vi "Robot Main.vi"() -> ()   [LabVIEW 2015]
doc: "Robot Main serves as the primary scheduler for your command and control robotics program. It should not be necessary to modify this VI. Instead, you should add your code to the VIs called from Robot Main - Teleop, Autonomous, and SubSystems."
uses:
  <vilib>/Rock Robotics/WPI/Camera/WPI_CameraImageSize.ctl
  Robot Type Def.ctl
  <vilib>/Rock Robotics/SystemInterfaces/NetworkCommunication/NetComm_UsageReport_ResourceType.ctl
  Framework/Robot Global Data.vi
  <vilib>/Rock Robotics/Network Tables/NT Write String.vi
panel:
  out "Application:Version Number":string
  in  "Time Stamp":timestamp
  out "Robot":T1=enum."Ghost"
  in  "error in":errorcluster
  in  "Enable LED Lights":bool
  in  "Image Size":T2=enum."320x240"
  in  "Enable Vision":bool
  in  "Finish":bool
  # "Make sure to set robot type"
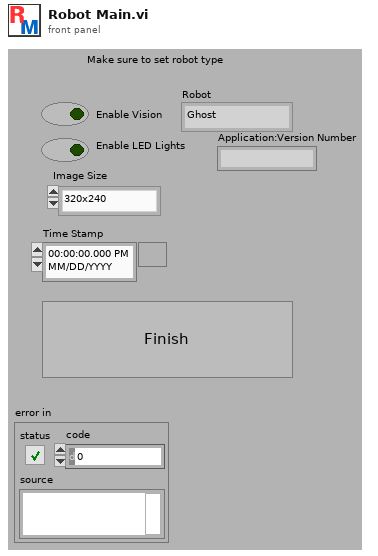
[diagram p1: front panel]
types:
  T1 = typedef "Robot Type Def.ctl" = enum32{"Disabled", "Ghost", "Casper", "Lofty", "Board", "RaceRobot"}
  T2 = typedef "WPI_CameraImageSize.ctl" = enum16{"640x480", "320x240", "160x120", "Custom"}
  T3 = typedef "NetComm_UsageReport_ResourceType.ctl" = enum8{"Controller", "Module", "Language", "CANPlugin", "Accelerometer", "ADXL345", "AnalogChannel", "AnalogTrigger", "AnalogTriggerOutput", "CANJaguar", "Compressor", "Counter", "Dashboard", "DigitalInput", "DigitalOutput", "DriverStationCIO", "DriverStationEIO", "DriverStationLCD", "Encoder", "GearTooth", "Gyro", "I2C", "Framework", "Jaguar", "Joystick", "Kinect", "KinectStick", "PIDController", "Preferences", "PWM", "Relay", "RobotDrive", "SerialPort", "Servo", "Solenoid", "SPI", "Task", "Ultrasonic", "Victor", "Button", "Command", "AxisCamera", "PCVideoServer", "SmartDashboard", "Talon", "HiTechnicColorSensor", "HiTechnicAccel", "HiTechnicCompass", "SRF08", "AnalogOutput", "Victor SP", "Talon SRX", "CAN Talon SRX", "ADXL362 Accel", "ADXRS450 Gyro", "Rev SPARK", "Mindsensors SD540", "Digital Filter"}
  T4 = typedef "WPI_DriverStationMatch Info.ctl" = cluster{"Autonomous Elapsed Seconds":dbl, "TeleOp Elapsed Seconds":dbl, "Disabled Elapsed Seconds":dbl, "Visited Autonomous":bool, "Visited TeleOp":bool, "Visited Disabled":bool, "Autonomous Settings":cluster{"Autonomous Style":enum16{"Iterative", "Independent"}, "VI Refnum":refnum<vi>}}
  T5 = typedef "WPI_DriverStationDerivedRobotMode.ctl" = enum16{"Init", "Execute", "Stop"}
  T6 = typedef "WPI_DriverStationRobotMode2.ctl" = enum16{"Autonomous Disabled", "Autonomous Enabled", "Teleop Disabled", "Teleop Enabled", "Disconnected", "Finish", "Test Disabled", "Test Enabled", "Emergency Stopped"}
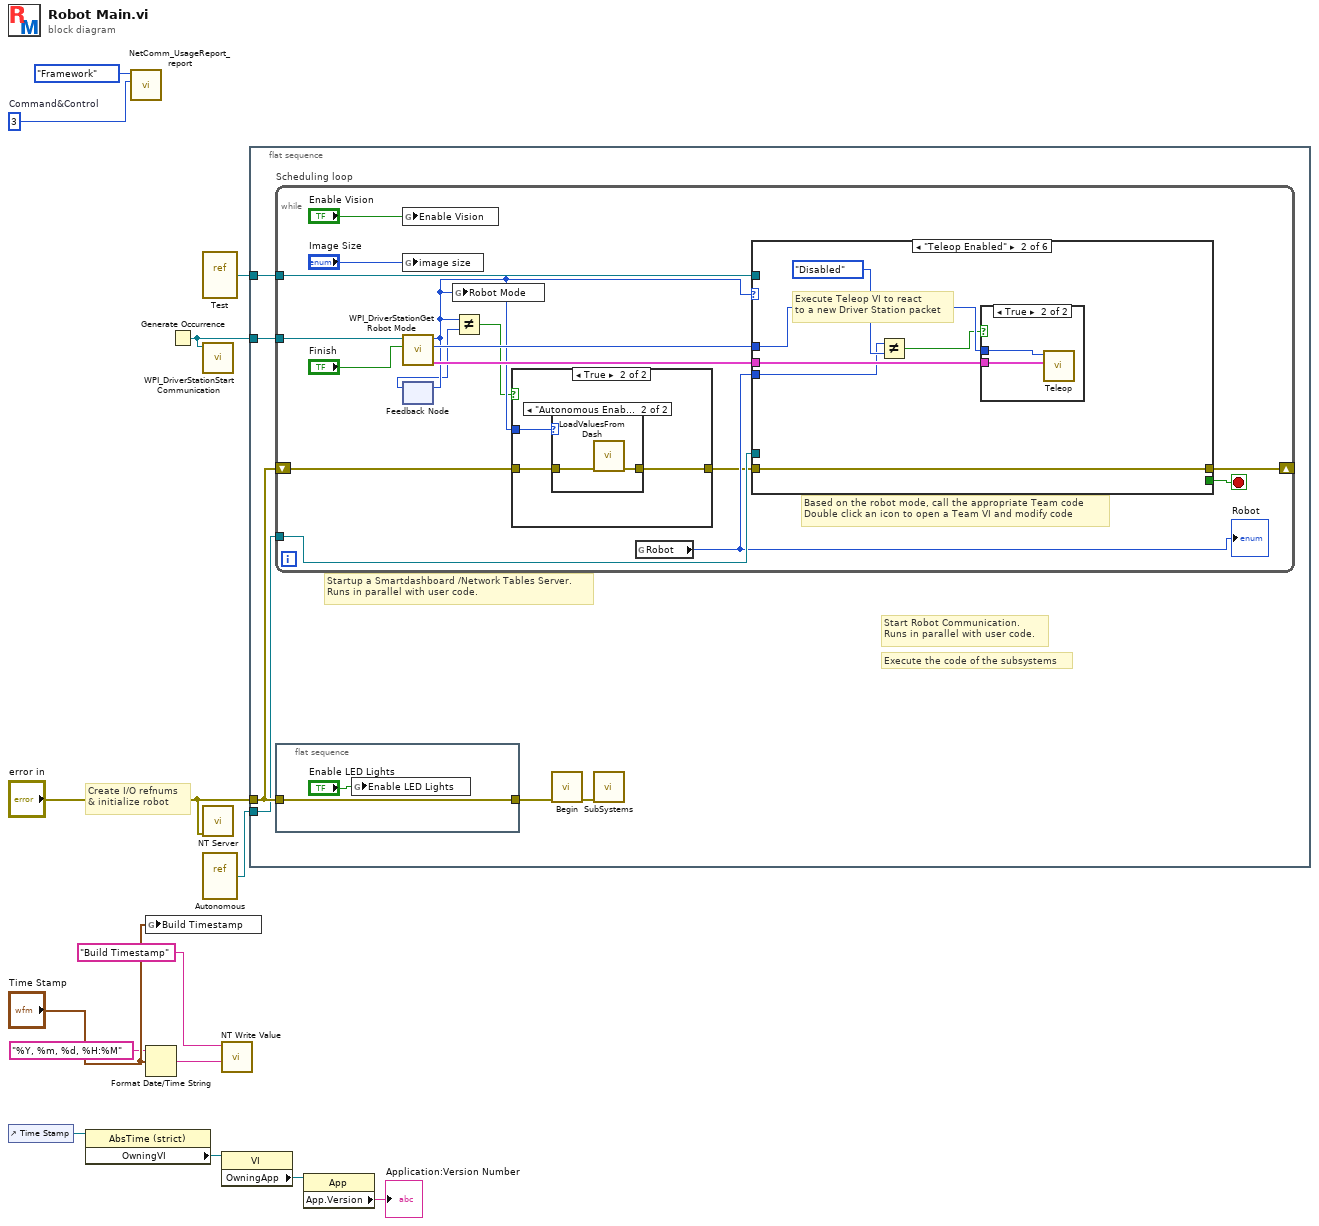
[diagram p0: block diagram]
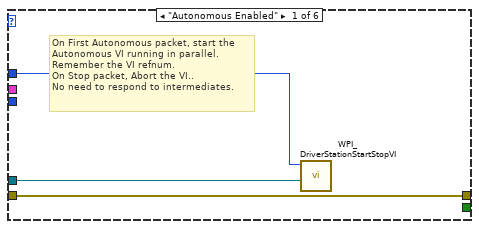
[diagram p4: hidden frame]
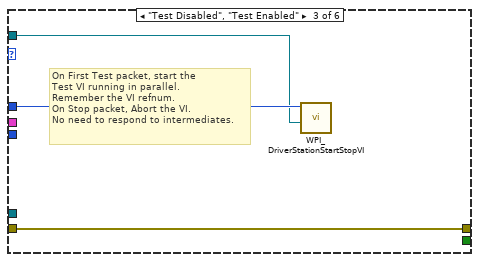
[diagram p6: hidden frame]
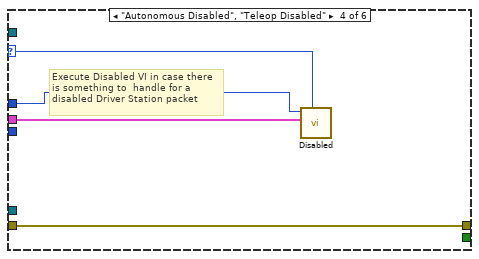
[diagram p7: hidden frame]
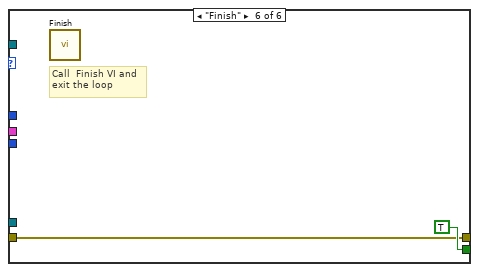
[diagram p9: hidden frame]
diagram:
  w9 = u8 3  # Command&Control
  # "Create I/O refnums\n& initialize robot"
  n1 = control-ref of="Time Stamp"() -> (w4:refnum<vi>)
  n2 = property class="AbsTime (strict)"(reference=w4) -> ("OwningVI"=w3:refnum<vi>)  [unwired: 1 in, 2 out]
  n3 = call <vilib>:"NetComm_UsageReport_report.vi"("Instance Number"=w9, "Resource Type"=NetComm_UsageReport_ResourceType."Framework") -> ()  [unwired: 10 in]
  n4 = global write "Robot Global Data.vi" "Build Timestamp"("Time Stamp") -> ()
  n5 = Format Date/Time String(time format string (%c)="%Y, %m, %d, %H:%M", seconds (now)="Time Stamp") -> (date/time string=w7:string)  [unwired: 1 in]
  n6 = Generate Occurrence() -> (w13:refnum<k4>)
  n7 = vi-ref "Test.vi"() -> (w11:refnum<vi>)
  n8 = call <vilib>:"WPI_DriverStationStart Communication.vi"("occurrence"=w13) -> ()  [unwired: 1 in, 10 out]
  n9 = call <vilib>:"NT Server.vi"("error in (no error)"="error in") -> ()  [unwired: 11 in]
  n10 = vi-ref "Autonomous.vi"() -> (w12:refnum<vi>)
  n11 = call-poly <vilib>:"NT Write Value.vi"("String"=w7, "Name"="Build Timestamp") -> ()  [unwired: 9 in, 1 out]
  n12 = property class="VI"(reference=w3) -> ("OwningApp"=w2:refnum<vi>)  [unwired: 1 in, 2 out]
  n13 = flat-sequence {
    tunnel: "error in" -> [w20]
    tunnel: w13 -> [w19]
    tunnel: w12 -> [w18]
    tunnel: w11 -> [w17]
    frame #0 {
      # "Startup a Smartdashboard /Network Tables Server.\nRuns in parallel with user code."
      # "Execute the code of the subsystems"
      # "Start Robot Communication.\nRuns in parallel with user code."
      n14 = while "Scheduling loop" {
        tunnel: w19 -> [w37]
        tunnel: w18 -> [w32]
        tunnel: w17 -> [w30]
        shift-right: [w23] -> _
        shift-left: w20 -> [w25]
        stop <- w34 stop-if-true
        # "Based on the robot mode, call the appropriate Team code\nDouble click an icon to open a Team VI and modify code"
        n15 = global write "Robot Global Data.vi" "Enable Vision"("Enable Vision") -> ()
        n16 = global write "Robot Global Data.vi" "image size"("Image Size") -> ()
        n17 = call <vilib>:"WPI_DriverStationGet Robot Mode.vi"("Finish"="Finish", "DS Occurrence"=w37) -> ("Match Info out"=w35:T4, "Call Context"=w38:T5, "Robot Mode"=w29:T6)  [unwired: 7 out]
        n18 = feedback-in #1(w29) -> ()
        n19 = feedback #1() -> (w28:T6)  [unwired: 1 in]
        n20 = global write "Robot Global Data.vi" "Robot Mode"(w29) -> ()
        n21 = Not Equal?(x=w29, y=w28) -> (x != y?=w27:bool)
        n22 = case shown="True" w27 {
          tunnel: w29 -> [_ w42]
          tunnel: w25 -> [w39 w41]
          tunnel: [w39 w40] -> w24
          frame False {
          }
          frame True {
            n23 = case shown="\"Autonomous Enabled\", \"Teleop Enabled\"" w42 {
              tunnel: w41 -> [w43 w45]
              tunnel: [w43 w44] -> w40
              frame Default {
              }
              frame "Autonomous Enabled", "Teleop Enabled" {
                n24 = call "LoadValuesFromDash.vi"("error in"=w45) -> ("error out"=w44:errorcluster)  [unwired: 10 in]
              }
            }
          }
        }
        n25 = global read "Robot Global Data.vi" "Robot"() -> (w26:T1)
        "Robot" <- w26
        n26 = case shown="\"Teleop Enabled\"" w29 {
          selector: w29 -> [_ _ _ w61 _ _]
          tunnel: w38 -> [w48 w54 w59 w63 _ _]
          tunnel: w35 -> [_ w53 _ w62 _ _]
          tunnel: [_ _ _ _ _ TRUE] -> w34
          tunnel: w32 -> [w47 _ _ _ _ _]
          tunnel: w30 -> [_ _ w58 _ _ _]
          tunnel: w26 -> [_ w50 _ _ _ _]
          tunnel: w24 -> [w46 w49 w57 w60 w64 w65]
          tunnel: [w46 w49 w57 w60 w64 w65] -> w23
          frame "Autonomous Enabled" {
            # "On First Autonomous packet, start the\nAutonomous VI running in parallel.\nRemember the VI refnum.\nOn Stop packet, Abort the VI..\nNo need to respond to intermediates."
            n27 = call <vilib>:"WPI_DriverStationStartStopVI.vi"("VI in"=w47, "Call Context"=w48) -> ()  [unwired: 10 in]
          }
          frame "Teleop Enabled" {
            # "Execute Teleop VI to react\nto a new Driver Station packet"
            n28 = Not Equal?(x=w50, y=Robot_Type_Def."Disabled" ("Robot")) -> (x != y?=w52:bool)
            n29 = case shown="True" w52 {
              tunnel: w54 -> [_ w56]
              tunnel: w53 -> [_ w55]
              frame False {
              }
              frame True {
                n30 = call "Teleop.vi"("Match Info"=w55, "Call Context"=w56) -> ()  [unwired: 1 in, 9 out]
              }
            }
          }
          frame "Test Disabled", "Test Enabled" {
            # "On First Test packet, start the\nTest VI running in parallel.\nRemember the VI refnum.\nOn Stop packet, Abort the VI.\nNo need to respond to intermediates."
            n31 = call <vilib>:"WPI_DriverStationStartStopVI.vi"("VI in"=w58, "Call Context"=w59) -> ()  [unwired: 10 in]
          }
          frame "Autonomous Disabled", "Teleop Disabled" {
            # "Execute Disabled VI in case there\nis something to  handle for a\ndisabled Driver Station packet"
            n32 = call "Disabled.vi"("Robot Mode"=w61, "Match Info"=w62, "Call Context"=w63) -> ()  [unwired: 1 in, 8 out]
          }
          frame "Disconnected", Default {
            # "Driver Station packet didn't arrive.\nPossibly useful for diagnostics"
          }
          frame "Finish" {
            # "Call  Finish VI and\nexit the loop"
            n33 = call "Finish.vi"() -> ()  [unwired: 1 in, 7 out]
          }
        }
      }
      n34 = flat-sequence {
        tunnel: w20 -> [w22]
        tunnel: [w22] -> w16
        frame #0 {
          n35 = global write "Robot Global Data.vi" "Enable LED Lights"("Enable LED Lights") -> ()
        }
      }
      n36 = call "Begin.vi"("error in"=w16) -> ("error out"=w15:errorcluster)  [unwired: 1 in, 9 out]
      n37 = call "SubSystems.vi"("error in"=w15) -> ()  [unwired: 11 in]
    }
  }
  n38 = property class="App"(reference=w2) -> ("App.Version"=→"Application:Version Number":string)  [unwired: 1 in, 2 out]
